vi "instrument_cluster.vi"() -> ()   [LabVIEW 2014]
uses:
  stateCtl.ctl
  <vilib>/Utility/miscctls.llb/LVTextColorsTypeDef.ctl
  <vilib>/Utility/miscctls.llb/LVSelectionTypeDef.ctl
  <vilib>/Utility/miscctls.llb/LVFontTypeDef.ctl
  <vilib>/Utility/miscctls.llb/LVForegroundBackgroundColorsTypeDef.ctl
  <vilib>/Instr/_visa.llb/VISA Configure Serial Port (Instr).vi
panel:
  out "Input String":string
  out "S5":string
  out "S4":string
  out "S3":string
  out "S2":string
  out "S1":string
  out "S0":string
  in  "Text.Font 4":T1={"Font Name"="Arial", "Size"=0, "Bold"=FALSE, "Italic"=FALSE, "Underline"=FALSE, "Strikeout"=FALSE, "Color"=16776746}
  in  "Text.Text Colors 2":T2={"Text Color"=0, "Background Color"=3153414}
  in  "Text.Selection 2":T3
  in  "Text.Font 2":T1={"Font Name"="Arial", "Size"=55, "Bold"=FALSE, "Italic"=FALSE, "Underline"=FALSE, "Strikeout"=FALSE, "Color"=16776746}
  in  "Text.Colors 2":T4={"Foreground Color"=0, "Background Color"=3153414}
  in  "Text.Text Colors 3":T2={"Text Color"=0, "Background Color"=3153414}
  in  "Text.Selection 3":T3
  in  "Text.Font 3":T1={"Font Name"="Arial", "Size"=0, "Bold"=FALSE, "Italic"=FALSE, "Underline"=FALSE, "Strikeout"=FALSE, "Color"=16776746}
  in  "Text.Colors 3":T4={"Foreground Color"=0, "Background Color"=3153414}
  in  "Text.Colors":T4={"Foreground Color"=0, "Background Color"=3153414}
  in  "Text.Font":T1={"Font Name"="Arial", "Size"=15, "Bold"=FALSE, "Italic"=FALSE, "Underline"=FALSE, "Strikeout"=FALSE, "Color"=16776746}
  in  "Text.Selection":T3
  in  "Text.Text Colors":T2={"Text Color"=0, "Background Color"=3153414}
  out "exitLed":bool
  out "statusBar":string="     "
  in  "startButton":bool
  out "stopLed":bool
  out "startLed":bool
  in  "VISA Serial Port":refnum<visa-resource-name>
  in  "exitButton":bool
  in  "stopButton":bool
  out "FE":string
  out "FP":string
  out "isRunning":bool
  out "state":T5=enum."exit"
  # "String G"
  # "Gear String"
  # "Travelled Distance String"
  # "Pedal Position String"
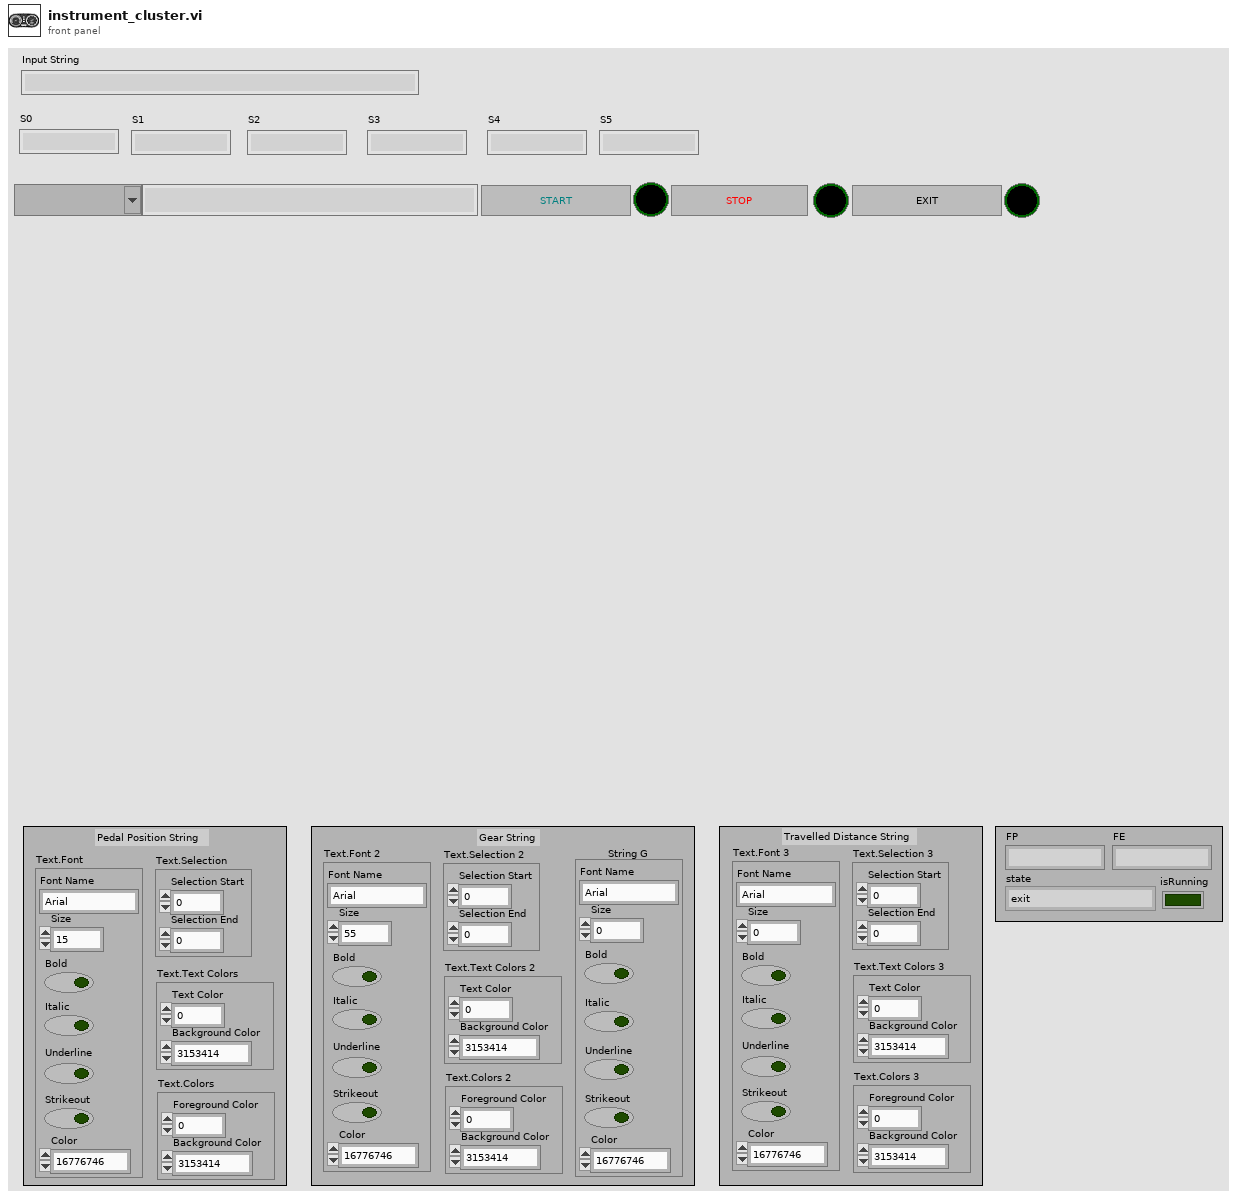
[diagram p1: front panel]
types:
  T1 = typedef "LVFontTypeDef.ctl" = cluster{"Font Name":string, "Size":u16, "Bold":bool, "Italic":bool, "Underline":bool, "Strikeout":bool, "Color":u32}
  T2 = typedef "LVTextColorsTypeDef.ctl" = cluster{"Text Color":u32, "Background Color":u32}
  T3 = typedef "LVSelectionTypeDef.ctl" = cluster{"Selection Start":u32, "Selection End":u32}
  T4 = typedef "LVForegroundBackgroundColorsTypeDef.ctl" = cluster{"Foreground Color":u32, "Background Color":u32}
  T5 = typedef "stateCtl.ctl" = enum16{"init", "ready", "running", "stopped", "exit"}
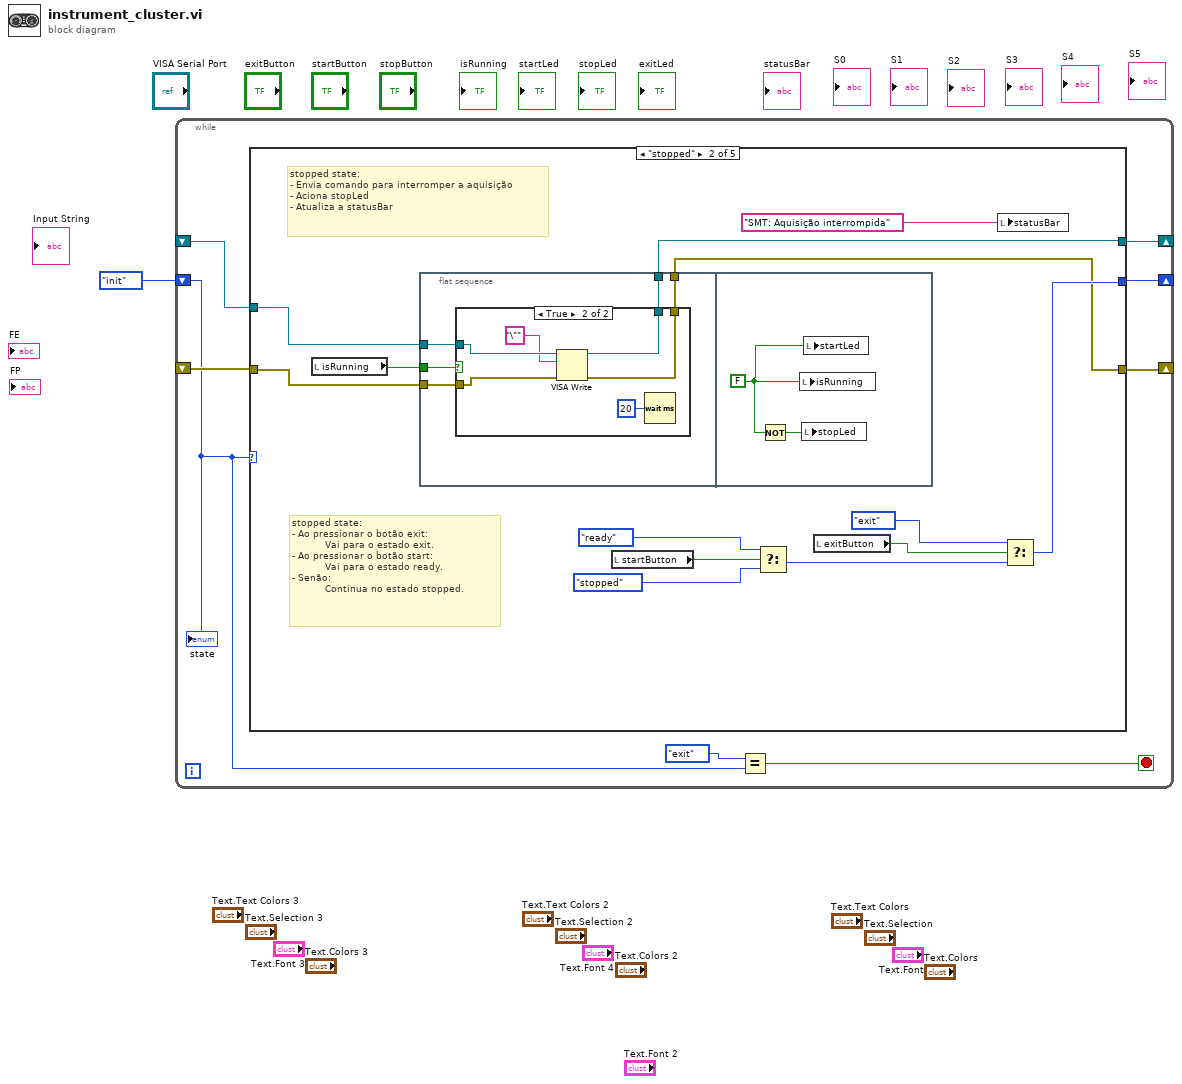
[diagram p0: block diagram]
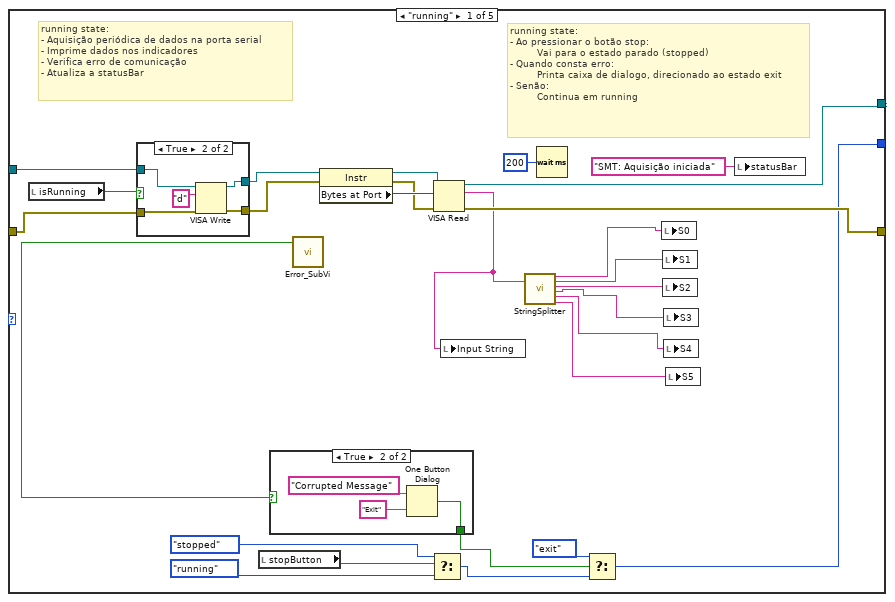
[diagram p2: hidden frame]
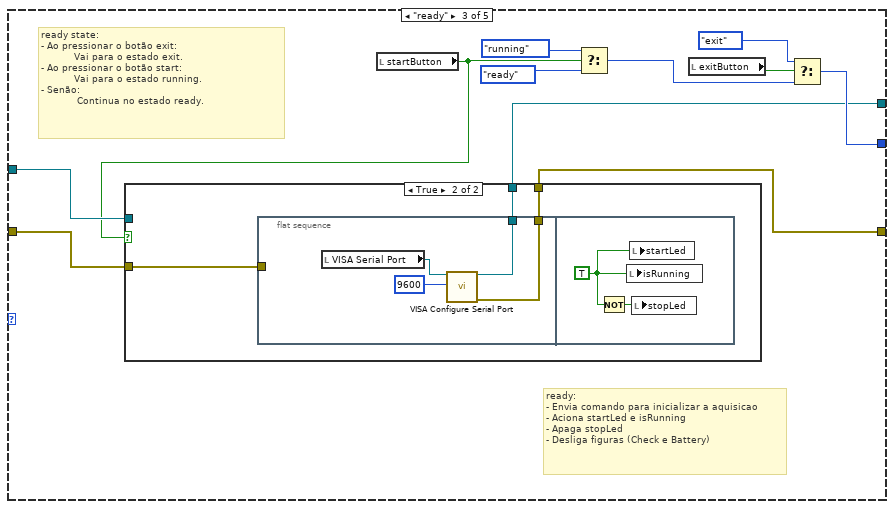
[diagram p6: hidden frame]
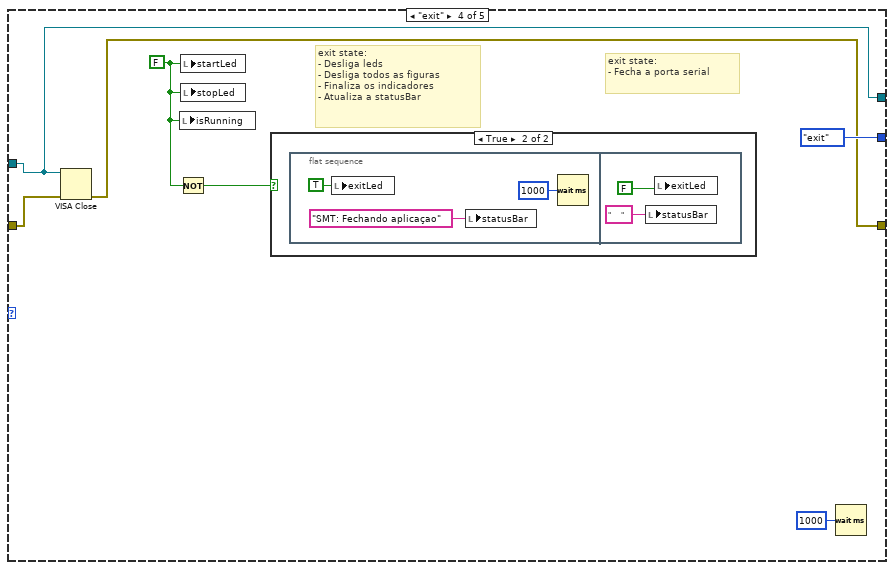
[diagram p8: hidden frame]
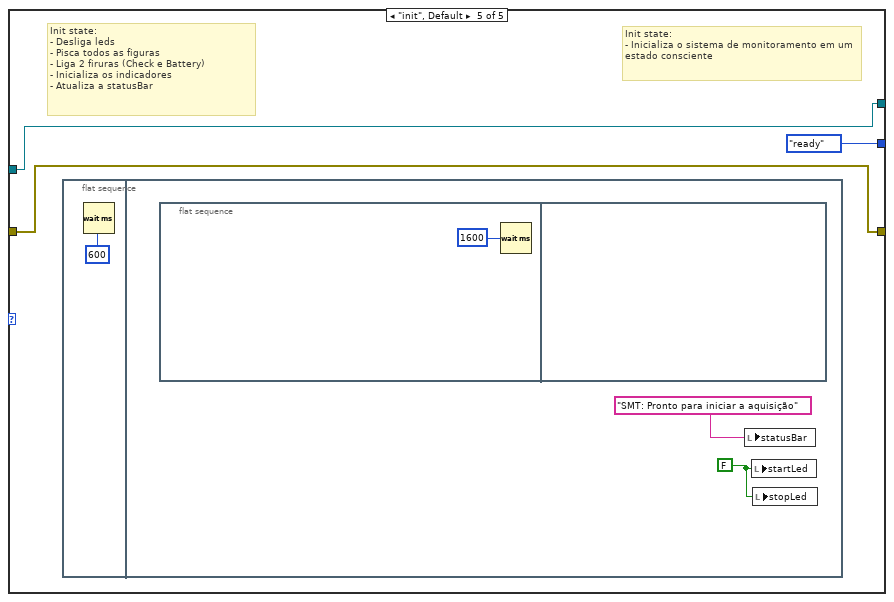
[diagram p10: hidden frame]
diagram:
  n1 = while {
    shift-right: [w3] -> _
    shift-left: _ -> [w8]
    shift-right: [w9] -> _
    shift-left: _ -> [w7]
    shift-right: [w4] -> _
    shift-left: stateCtl."init" ("state") -> [w5]
    stop <- w2 stop-if-true
    n2 = case shown="\"stopped\"" w5 {
      tunnel: [w29 w52 w78 w101 w111] -> w3
      tunnel: [w28 w53 w77 w102 w110] -> w9
      tunnel: [w21 w58 w81 stateCtl."exit" ("state") stateCtl."ready" ("state")] -> w4
      tunnel: w8 -> [w23 w56 w79 w101 w111]
      tunnel: w7 -> [w24 w55 w80 w103 w110]
      frame "running" {
        # "running state:\n- Ao pressionar o botão stop: \n         Vai para o estado parado (stopped)\n- Quando consta erro:\n         Printa caixa de dialogo, direcionado ao estado exit  \n- Senão:          \n         Continua em running"
        # "running state:\n- Aquisição periódica de dados na porta serial\n- Imprime dados nos indicadores\n- Verifica erro de comunicação\n- Atualiza a statusBar"
        n3 = local read "isRunning"() -> (w18:bool)
        n4 = case shown="True" w18 {
          tunnel: [w42 w46] -> w26
          tunnel: [w41 w45] -> w25
          tunnel: w24 -> [w42 w44]
          tunnel: w23 -> [w41 w43]
          frame False {
          }
          frame True {
            n5 = VISA Write(VISA resource name=w43, write buffer="d", error in (no error)=w44) -> (VISA resource name out=w45:refnum<visa-resource-name>, error out=w46:errorcluster)  [unwired: 1 out]
          }
        }
        n6 = local read "stopButton"() -> (w34:bool)
        n7 = call "Error_SubVi.vi"() -> ("error"=w17:bool)  [unwired: 11 in]
        n8 = case shown="True" w17 {
          selector: w17 -> [w37 _]
          tunnel: [w37 w38] -> w19
          frame False {
          }
          frame True {
            n9 = One Button Dialog(message="Corrupted Message", button name ("OK")="Exit") -> (true=w38:bool)
          }
        }
        n10 = property class="Instr"(reference=w25, error in=w26) -> (reference out=w30:refnum<visa-resource-name>, error out=w31:errorcluster, "Bytes at Port"=w32:u32)
        n11 = Select(t=stateCtl."stopped" ("state"), s=w34, f=stateCtl."running" ("state")) -> (s? t:f=w20:T5)
        n12 = VISA Read(VISA resource name=w30, byte count=w32, error in (no error)=w31) -> (VISA resource name out=w29:refnum<visa-resource-name>, read buffer=w10:string, error out=w28:errorcluster)  [unwired: 1 out]
        n13 = local write "Input String"(w10) -> ()
        n14 = call "StringSplitter.vi"("Input String"=w10) -> ("S0"=w16:string, "S1"=w15:string, "S2"=w14:string, "S3"=w13:string, "S4"=w12:string, "S5"=w11:string)  [unwired: 13 in]
        n15 = Wait (ms)(milliseconds to wait=u32 200) -> ()  [unwired: 1 out]
        n16 = Select(t=stateCtl."exit" ("state"), s=w19, f=w20) -> (s? t:f=w21:T5)
        n17 = local write "S0"(w16) -> ()
        n18 = local write "S1"(w15) -> ()
        n19 = local write "S2"(w14) -> ()
        n20 = local write "S3"(w13) -> ()
        n21 = local write "S4"(w12) -> ()
        n22 = local write "S5"(w11) -> ()
        n23 = local write "statusBar"("SMT: Aquisição iniciada" ("statusBar")) -> ()
      }
      frame "stopped" {
        # "stopped state:\n- Ao pressionar o botão exit: \n           Vai para o estado exit.\n- Ao pressionar o botão start:\n           Vai para o estado ready.\n- Senão:\n           Continua no estado stopped."
        # "stopped state:\n- Envia comando para interromper a aquisição\n- Aciona stopLed\n- Atualiza a statusBar"
        n24 = local read "isRunning"() -> (w54:bool)
        n25 = flat-sequence {
          tunnel: w56 -> [w65]
          tunnel: w55 -> [w64]
          tunnel: w54 -> [w63]
          tunnel: [w62] -> w53
          tunnel: [w61] -> w52
          frame #0 {
            n26 = case shown="True" w63 {
              tunnel: w65 -> [w67 w73]
              tunnel: w64 -> [w66 w72]
              tunnel: [w66 w68] -> w62
              tunnel: [w67 w70] -> w61
              frame False {
              }
              frame True {
                n27 = VISA Write(VISA resource name=w73, write buffer="\"", error in (no error)=w72) -> (VISA resource name out=w70:refnum<visa-resource-name>, error out=w68:errorcluster)  [unwired: 1 out]
                n28 = Wait (ms)(milliseconds to wait=u32 20) -> ()  [unwired: 1 out]
              }
            }
          }
          frame #1 {
            w75 = FALSE ("Boolean")
            n29 = Not(x=w75) -> (.not. x?=w74:bool)
            n30 = local write "isRunning"(w75) -> ()
            n31 = local write "stopLed"(w74) -> ()
            n32 = local write "startLed"(w75) -> ()
          }
        }
        n33 = local read "startButton"() -> (w51:bool)
        n34 = Select(t=stateCtl."ready" ("state"), s=w51, f=stateCtl."stopped" ("state")) -> (s? t:f=w59:T5)
        n35 = local read "exitButton"() -> (w50:bool)
        n36 = local write "statusBar"("SMT: Aquisição interrompida" ("statusBar")) -> ()
        n37 = Select(t=stateCtl."exit" ("state"), s=w50, f=w59) -> (s? t:f=w58:T5)
      }
      frame "ready" {
        # "ready state:\n- Ao pressionar o botão exit: \n           Vai para o estado exit.\n- Ao pressionar o botão start:\n           Vai para o estado running.\n- Senão:\n            Continua no estado ready."
        # "ready:\n- Envia comando para inicializar a aquisicao\n- Aciona startLed e isRunning\n- Apaga stopLed\n- Desliga figuras (Check e Battery)"
        n38 = local read "startButton"() -> (w76:bool)
        n39 = case shown="True" w76 {
          tunnel: [w88 w89] -> w78
          tunnel: [w87 w90] -> w77
          tunnel: w79 -> [w88 _]
          tunnel: w80 -> [w87 w91]
          frame False {
          }
          frame True {
            n40 = flat-sequence {
              tunnel: w91 -> [_]
              tunnel: [w93] -> w90
              tunnel: [w92] -> w89
              frame #0 {
                n41 = local read "VISA Serial Port"() -> (w94:refnum<visa-resource-name>)
                n42 = call-poly "VISA Configure Serial Port"("VISA resource name"=w94, "baud rate (9600)"=u32 9600) -> ("VISA resource name out"=w92:refnum<visa-resource-name>, "error out"=w93:errorcluster)  [unwired: 12 in]
              }
              frame #1 {
                w97 = TRUE ("Boolean")
                n43 = Not(x=w97) -> (.not. x?=w96:bool)
                n44 = local write "isRunning"(w97) -> ()
                n45 = local write "startLed"(w97) -> ()
                n46 = local write "stopLed"(w96) -> ()
              }
            }
          }
        }
        n47 = Select(t=stateCtl."running" ("state"), s=w76, f=stateCtl."ready" ("state")) -> (s? t:f=w82:T5)
        n48 = local read "exitButton"() -> (w84:bool)
        n49 = Select(t=stateCtl."exit" ("state"), s=w84, f=w82) -> (s? t:f=w81:T5)
      }
      frame "exit" {
        w99 = FALSE ("startLed")
        # "exit state:\n- Desliga leds\n- Desliga todos as figuras\n- Finaliza os indicadores\n- Atualiza a statusBar"
        # "exit state:\n- Fecha a porta serial"
        n50 = VISA Close(VISA resource name=w101, error in (no error)=w103) -> (error out=w102:errorcluster)
        n51 = Not(x=w99) -> (.not. x?=w100:bool)
        n52 = local write "isRunning"(w99) -> ()
        n53 = local write "startLed"(w99) -> ()
        n54 = local write "stopLed"(w99) -> ()
        n55 = case shown="True" w100 {
          frame False {
          }
          frame True {
            n56 = flat-sequence {
              frame #0 {
                n57 = local write "exitLed"(TRUE ("exitLed")) -> ()
                n58 = local write "statusBar"("SMT: Fechando aplicaçao" ("statusBar")) -> ()
                n59 = Wait (ms)(milliseconds to wait=u32 1000) -> ()  [unwired: 1 out]
              }
              frame #1 {
                n60 = local write "statusBar"("     " ("statusBar")) -> ()
                n61 = local write "exitLed"(FALSE ("exitLed")) -> ()
              }
            }
          }
        }
        n62 = Wait (ms)(milliseconds to wait=u32 1000) -> ()  [unwired: 1 out]
      }
      frame "init", Default {
        # "Init state:\n- Inicializa o sistema de monitoramento em um estado consciente"
        # "Init state:\n- Desliga leds\n- Pisca todos as figuras\n- Liga 2 firuras (Check e Battery)\n- Inicializa os indicadores\n- Atualiza a statusBar"
        n63 = flat-sequence {
          frame #0 {
            n64 = Wait (ms)(milliseconds to wait=u32 600) -> ()  [unwired: 1 out]
          }
          frame #1 {
            w115 = FALSE
            n65 = flat-sequence {
              frame #0 {
                n66 = Wait (ms)(milliseconds to wait=u32 1600) -> ()  [unwired: 1 out]
              }
              frame #1 {
              }
            }
            n67 = local write "statusBar"("SMT: Pronto para iniciar a aquisição" ("statusBar")) -> ()
            n68 = local write "startLed"(w115) -> ()
            n69 = local write "stopLed"(w115) -> ()
          }
        }
      }
    }
    n70 = Equal?(x=stateCtl."exit" ("state"), y=w5) -> (x = y?=w2:bool)
    "state" <- w5
  }
